vi "Delete String Array Element.vi"(10 "Element to Delete":string, 11 "Array in":string[](array[string])) -> (2 "Found and Deleted":bool, 3 "Array out":string[](array[string]))   [LabVIEW 2020, in "Wordle Engine.lvlib"]
uses:
  Wordle Engine.lvlib
  fe6ff793-1998-4283-98d7-6c1f135b3a18.vi/d4db2432-cc9c-482c-8957-dac855435ef6.vi
  fe6ff793-1998-4283-98d7-6c1f135b3a18.vi/86fbf154-bd7b-49a2-8ab2-a837b2a95f24.vi
  fe6ff793-1998-4283-98d7-6c1f135b3a18.vi/3b95b01e-1ec2-4565-bcd9-7606a5281010.vi
  fe6ff793-1998-4283-98d7-6c1f135b3a18.vi/96a08935-737a-44b2-979c-a81d56408f7e.vi
  fe6ff793-1998-4283-98d7-6c1f135b3a18.vi/d4db2432-cc9c-482c-8957-dac855435ef6.vi/6eaecd13-6e48-4772-a921-b51ebdf84d88.vi
  fe6ff793-1998-4283-98d7-6c1f135b3a18.vi/d4db2432-cc9c-482c-8957-dac855435ef6.vi/d2d5f2b7-06f4-47f6-971c-049c3fdbb653.vi
  fe6ff793-1998-4283-98d7-6c1f135b3a18.vi/3b95b01e-1ec2-4565-bcd9-7606a5281010.vi/6eaecd13-6e48-4772-a921-b51ebdf84d88.vi
  fe6ff793-1998-4283-98d7-6c1f135b3a18.vi/3b95b01e-1ec2-4565-bcd9-7606a5281010.vi/d2d5f2b7-06f4-47f6-971c-049c3fdbb653.vi
  fe6ff793-1998-4283-98d7-6c1f135b3a18.vi/96a08935-737a-44b2-979c-a81d56408f7e.vi/6eaecd13-6e48-4772-a921-b51ebdf84d88.vi
  fe6ff793-1998-4283-98d7-6c1f135b3a18.vi/96a08935-737a-44b2-979c-a81d56408f7e.vi/d2d5f2b7-06f4-47f6-971c-049c3fdbb653.vi
  <vilib>/Comparison/Less/Less Functor/Less Functor.lvclass
  34fb09ad-82f2-4cc4-b24e-fe1593a329b2.vi
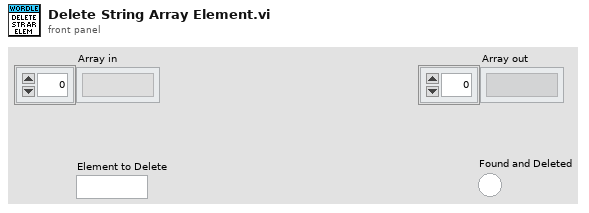
[diagram p1: front panel]
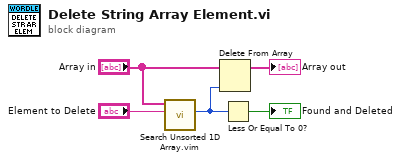
[diagram p0: block diagram]
diagram:
  n1 = call "Search Unsorted 1D Array.vim"("element"="Element to Delete", "unsorted 1D array"="Array in") -> ("index of element"=w2:i32)  [unwired: 9 in]
  n2 = Delete From Array(array="Array in", index=w2) -> (array with subset deleted=→"Array out":string[])  [unwired: 1 in, 1 out]
  n3 = Less Or Equal To 0?(x=w2) -> (x <= 0?=→"Found and Deleted":bool)
